vi "Contour Line.vi"   [LabVIEW 2017, in "NI_AAL_Geometry.lvlib"]
doc: "Calculates and returns the contour lines of a surface and the contour graph."
uses:
  <vilib>/Analysis/NI_AAL_Geometry.lvlib
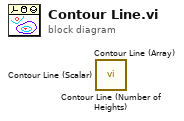
[diagram p0: block diagram]
diagram:
  n1 = call <vilib>:"Contour Line (Number of Heights).vi"() -> ()  [unwired: 9 in, 3 out]
  n2 = call <vilib>:"Contour Line (Array).vi"() -> ()  [unwired: 9 in, 3 out]
  n3 = call <vilib>:"Contour Line (Scalar).vi"() -> ()  [unwired: 9 in, 3 out]
